vi "Init.vi"(8 "error in (no error)":errorcluster, 10 "Params":variant, 11 "DAQmx Base in":refnum<class "NI DAQmx Base.lvclass">) -> (0 "error out":errorcluster, 3 "DAQmx Base out":refnum<class "NI DAQmx Base.lvclass">)   [LabVIEW 2020, in "NI DAQmx.lvlib" / "NI DAQmx Base.lvclass"]
uses:
  NI DAQmx Base.lvclass
  NI DAQmx Base.lvclass/NI DAQmx Base.ctl
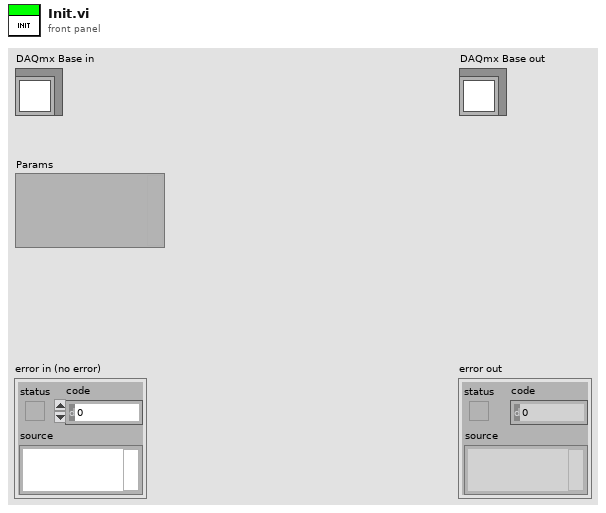
[diagram p1: front panel]
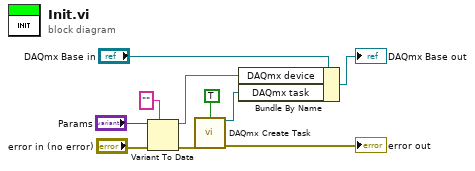
[diagram p0: block diagram]
diagram:
  n1 = Variant To Data(error in="error in (no error)", type="", Variant="Params") -> (data=w1:string, error out=w4:errorcluster)
  n2 = call <vilib>:"DAQmx Create Task.vi"("auto cleanup"=TRUE, "error in"=w4) -> ("task out"=w6:refnum<k21>, "error out"=→"error out":errorcluster)  [unwired: 12 in]
  n3 = Bundle By Name(cluster="DAQmx Base in", "DAQmx device"=w1, "DAQmx task"=w6) -> (→"DAQmx Base out":refnum<class "NI DAQmx Base.lvclass">)
